vi "Calculate Average.vi"(0 "Measurements":dbl[](array[numeric]), 5 "Aperture Time":dbl) -> (4 "Average level":dbl)   [LabVIEW 2024, in "devicePowerSequencerCoreLogic.lvlib"]
uses:
  devicePowerSequencerCoreLogic.lvlib
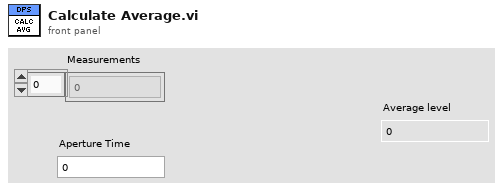
[diagram p1: front panel]
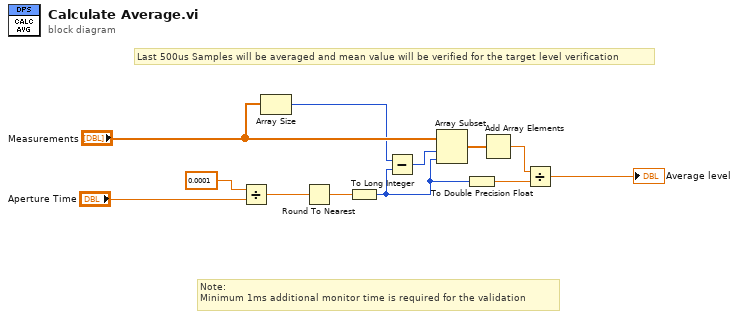
[diagram p0: block diagram]
diagram:
  # "Last 500us Samples will be averaged and mean value will be verified for the target level verification"
  # "Note:\nMinimum 1ms additional monitor time is required for the validation"
  n1 = Divide(x=0.0001, y="Aperture Time") -> (x/y=w8:dbl)
  n2 = Array Size(array="Measurements") -> (size(s)=w6:i32)
  n3 = Round To Nearest(number=w8) -> (nearest integer value=w7:dbl)
  n4 = To Long Integer(number=w7) -> (32bit integer=w2:i32)
  n5 = Subtract(x=w6, y=w2) -> (x-y=w5:i32)
  n6 = Array Subset(array="Measurements", index=w5, length=w2) -> (w4:dbl[])
  n7 = To Double Precision Float(number=w2) -> (double precision float=w1:dbl)
  n8 = Add Array Elements(numeric array=w4) -> (sum=w3:dbl)
  n9 = Divide(x=w3, y=w1) -> (x/y=→"Average level":dbl)
